vi "Find Size.vi"(8 "error in (no error)":errorcluster, 10 "p":i32, 11 "TeamEffort in":refnum<class "TeamEffort.lvclass">) -> (0 "error out":errorcluster, 3 "TeamEffort out":refnum<class "TeamEffort.lvclass">)   [LabVIEW 2015, in "TeamEffort.lvclass"]
uses:
  TeamEffort.lvclass
panel:
  in  "Maze (0: Empty, -1: Enemy. >0: Teammate":i32[][](array[numeric])
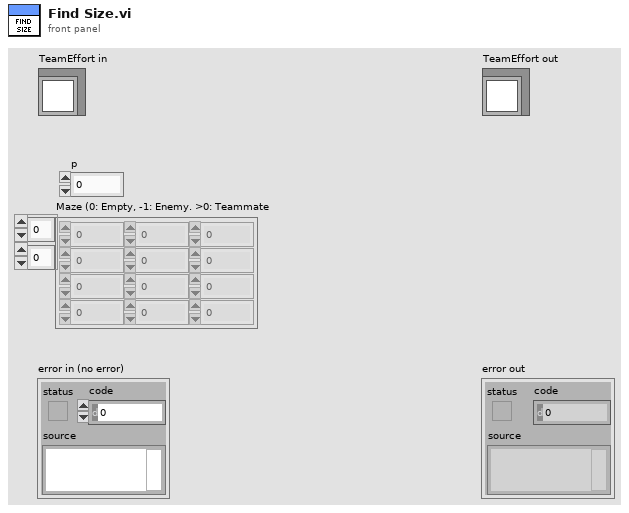
[diagram p1: front panel]
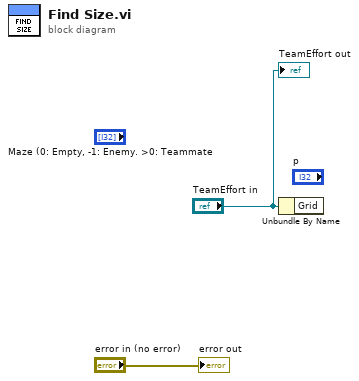
[diagram p0: block diagram]
diagram:
  n1 = Unbundle By Name("TeamEffort in") -> ()  [unwired: 1 out]
  "error out" <- "error in (no error)"
  "TeamEffort out" <- "TeamEffort in"
